vi "KListbox Test.vi"() -> ()   [LabVIEW 2015]
uses:
  KListbox.xctl
panel:
  out "KListbox 2":cluster{"Row":i32, "Items":string[]}(xcontrol)
  in  "stop":bool
  in  "KListbox":cluster{"Row":i32, "Items":string[]}(xcontrol)
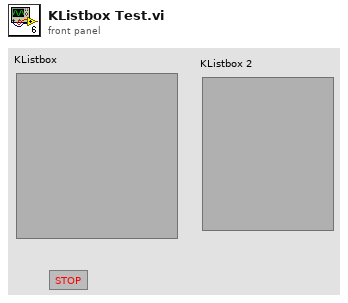
[diagram p1: front panel]
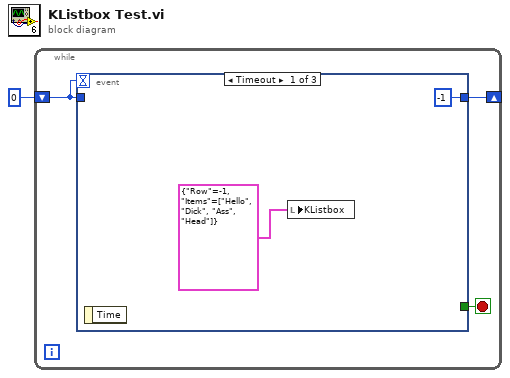
[diagram p0: block diagram]
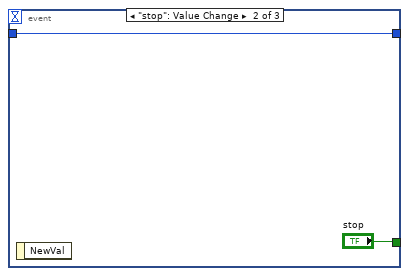
[diagram p2: hidden frame]
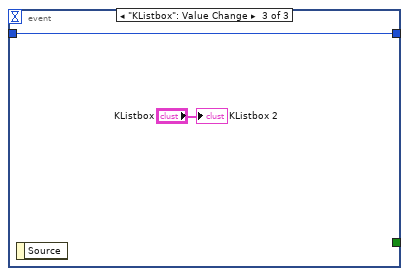
[diagram p3: hidden frame]
diagram:
  n1 = while {
    shift-right: [w2] -> _
    shift-left: 0 -> [w3]
    stop <- w4 stop-if-true
    n2 = event shown="[0] Timeout" {
      selector: _ -> [_ _ _]
      dyn-events: _ -> [_ _ _]
      timeout: w3 -> [_ _ _]
      tunnel: [_ "stop" _] -> w4
      tunnel: w3 -> [_ w7 w10]
      tunnel: [-1 w7 w10] -> w2
      event Timeout {
        n3 = event-data() -> ()  [unwired: 1 in, 1 out]
        n4 = local write "KListbox"(cluster{"Row":i32, "Items":string[]} {"Row"=-1, "Items"=["Hello", "Dick", "Ass", "Head"]} ("KListbox")) -> ()
      }
      event "stop": Value Change {
        n5 = event-data() -> ()  [unwired: 1 in, 1 out]
      }
      event "KListbox": Value Change {
        n6 = event-data() -> ()  [unwired: 1 in, 1 out]
        "KListbox 2" <- "KListbox"
      }
    }
  }
